vi "SignalCalculations.vi"(6 "Ref?":bool, 10 "MomentValues in":T1, 11 "All Data":dbl[][](array[numeric])) -> (2 "MomentValues Out":T1, 3 "Poperties":T2)   [LabVIEW 2019]
uses:
  Communication/TypeDef/#TypeDef_PropertiesToSave.ctl
  TypeDef/#TypeDef_MomentValues.ctl
  <vilib>/Analysis/5stat.llb/RMS (DBL).vi
  <vilib>/Analysis/NI_AALPro.lvlib
panel:
  out "size(s)":i32[](array[numeric])
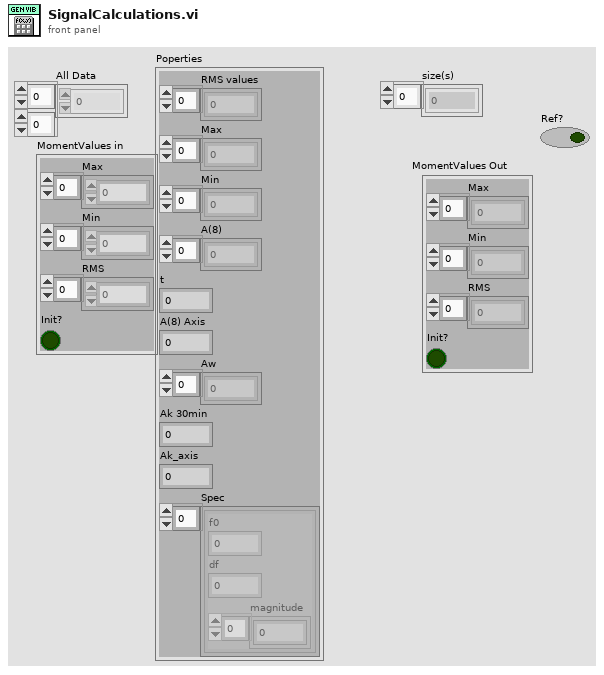
[diagram p1: front panel]
types:
  T1 = typedef "#TypeDef_MomentValues.ctl" = cluster{"Max":dbl[], "Min":dbl[], "RMS":dbl[], "Init?":bool}
  T2 = typedef "#TypeDef_PropertiesToSave.ctl" = cluster{"RMS values":dbl[], "Max":dbl[], "Min":dbl[], "A(8)":dbl[], "t":dbl, "A(8) Axis":dbl, "Aw":dbl[], "Ak 30min":dbl, "Ak_axis":i32, "Spec":cluster{"f0":dbl, "df":dbl, "magnitude":dbl[]}[]}
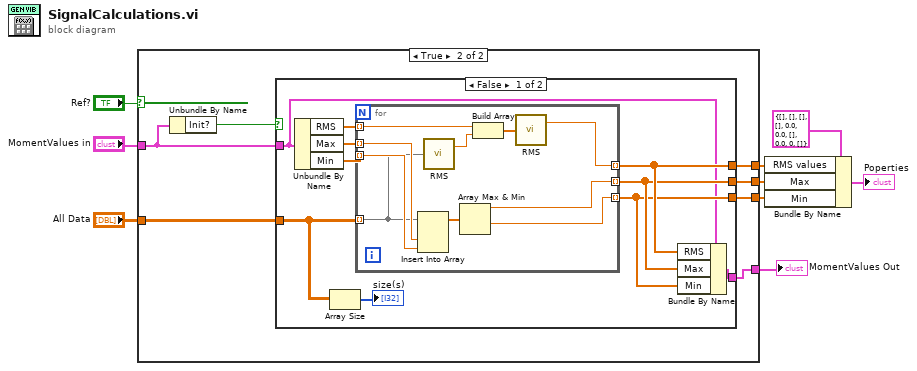
[diagram p0: block diagram]
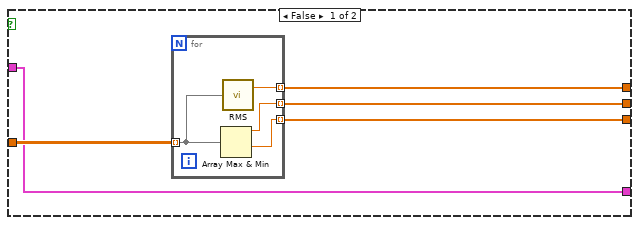
[diagram p2: hidden frame]
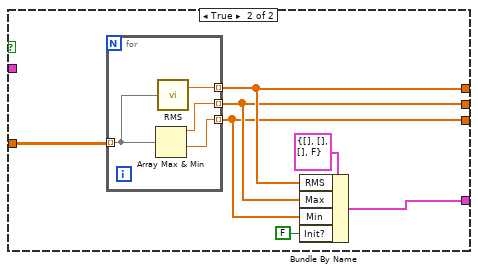
[diagram p3: hidden frame]
diagram:
  n1 = case shown="True" "Ref?" {
    tunnel: "All Data" -> [w14 w21]
    tunnel: [w13 w25] -> w6
    tunnel: [w12 w24] -> w5
    tunnel: [w11 w23] -> w4
    tunnel: "MomentValues in" -> [w10 w20]
    tunnel: [w10 w22] -> w3
    frame False {
      n2 = for {
        tunnel: w14 -> [w18] mode=indexing
        tunnel: [w17] -> w13 mode=indexing
        tunnel: [w16] -> w12 mode=indexing
        tunnel: [w15] -> w11 mode=indexing
        n3 = Array Max & Min(array=w18) -> (max value=w16:dbl, min value=w15:dbl)  [unwired: 2 out]
        n4 = call-poly <vilib>:"RMS.vi"("X"=w18) -> ("rms value"=w17:dbl)  [unwired: 1 out]
      }
    }
    frame True {
      n5 = Unbundle By Name(w20) -> ("Init?"=w19:bool)
      n6 = case shown="False" w19 {
        tunnel: [w32 w50] -> w25
        tunnel: [w31 w48] -> w24
        tunnel: [w30 w47] -> w23
        tunnel: w20 -> [w26 _]
        tunnel: [w29 w49] -> w22
        tunnel: w21 -> [w28 w51]
        frame False {
          n7 = Unbundle By Name(w26) -> ("RMS"=w33:dbl[], "Max"=w35:dbl[], "Min"=w34:dbl[])
          n8 = Array Size(array=w28) -> (size(s)=→"size(s)":i32[])
          n9 = for {
            tunnel: w35 -> [w45] mode=indexing
            tunnel: w34 -> [w44] mode=indexing
            tunnel: w28 -> [w40] mode=indexing
            tunnel: [w42] -> w31 mode=indexing
            tunnel: [w41] -> w30 mode=indexing
            tunnel: w33 -> [w39] mode=indexing
            tunnel: [w36] -> w32 mode=indexing
            n10 = Insert Into Array(array=w40, new element #1=w45, new element #2=w44) -> (w43:dbl[])  [unwired: 1 in]
            n11 = call-poly <vilib>:"RMS.vi"("X"=w40) -> ("rms value"=w38:dbl)  [unwired: 1 out]
            n12 = Array Max & Min(array=w43) -> (max value=w42:dbl, min value=w41:dbl)  [unwired: 2 out]
            n13 = Build Array(w39, w38) -> (w37:dbl[])
            n14 = call-poly <vilib>:"RMS.vi"("X"=w37) -> ("rms value"=w36:dbl)  [unwired: 1 out]
          }
          n15 = Bundle By Name(cluster=w26, "RMS"=w32, "Max"=w31, "Min"=w30) -> (w29:T1)
        }
        frame True {
          n16 = for {
            tunnel: w51 -> [w56] mode=indexing
            tunnel: [w55] -> w50 mode=indexing
            tunnel: [w54] -> w48 mode=indexing
            tunnel: [w53] -> w47 mode=indexing
            n17 = Array Max & Min(array=w56) -> (max value=w54:dbl, min value=w53:dbl)  [unwired: 2 out]
            n18 = call-poly <vilib>:"RMS.vi"("X"=w56) -> ("rms value"=w55:dbl)  [unwired: 1 out]
          }
          n19 = Bundle By Name(cluster=T1 {"Max"=[], "Min"=[], "RMS"=[], "Init?"=FALSE} ("MomentValues Out"), "RMS"=w50, "Max"=w48, "Min"=w47, "Init?"=FALSE) -> (w49:T1)
        }
      }
    }
  }
  "MomentValues Out" <- w3
  n20 = Bundle By Name(cluster=T2 {"RMS values"=[], "Max"=[], "Min"=[], "A(8)"=[], "t"=0.0, "A(8) Axis"=0.0, "Aw"=[], "Ak 30min"=0.0, "Ak_axis"=0, "Spec"=[]} ("Properties"), "RMS values"=w6, "Max"=w5, "Min"=w4) -> (→"Poperties":T2)
